vi "Write Data.vi"(8 "error in (no error)":errorcluster, 9 "Qsp":sgl, 10 "Q":sgl, 11 "AlicatVData in":refnum<class "AlicatVCData.lvclass">) -> (0 "error out":errorcluster, 3 "AlicatVData out":refnum<class "AlicatVCData.lvclass">)   [LabVIEW 2014, in "Alicat.lvlib" / "AlicatVCData.lvclass"]
uses:
  AlicatVCData.lvclass
  AlicatVCData.lvclass/AlicatVCData.ctl
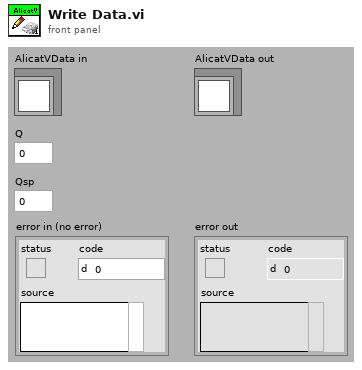
[diagram p1: front panel]
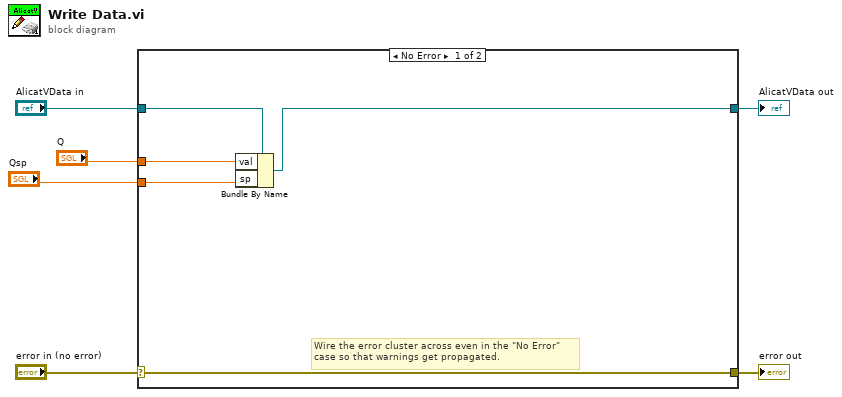
[diagram p0: block diagram]
diagram:
  n1 = case shown="No Error" "error in (no error)" {
    selector: "error in (no error)" -> [w11 w13]
    tunnel: [w11 w13] -> w5
    tunnel: [w7 w12] -> w3
    tunnel: "AlicatVData in" -> [w10 w12]
    tunnel: "Q" -> [w9 _]
    tunnel: "Qsp" -> [w8 _]
    frame No Error {
      # "Wire the error cluster across even in the \"No Error\"\ncase so that warnings get propagated."
      n2 = Bundle By Name(cluster=w10, "val"=w9, "sp"=w8) -> (w7:refnum<class "AlicatVCData.lvclass">)
    }
    frame Error {
    }
  }
  "error out" <- w5
  "AlicatVData out" <- w3
